vi "TimeTracker_GV.vi"(1 "Action":T1, 2 "Element In":T2) -> (6 "Elements Out":T2[](array[typedef]))   [LabVIEW 2014]
uses:
  Element.ctl
  States.ctl
panel:
  out "Init?":bool
  out "Error Out":errorcluster
  in  "Error In":errorcluster
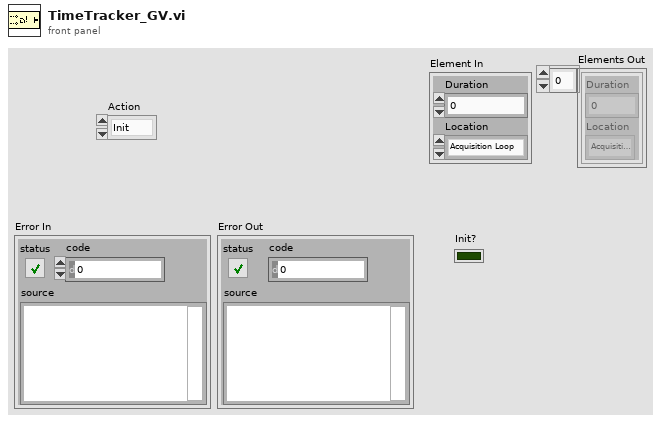
[diagram p1: front panel]
types:
  T1 = typedef "States.ctl" = enum16{"Init", "Flush", "Add"}
  T2 = typedef "Element.ctl" = cluster{"Duration":dbl, "Location":enum16{"Acquisition Loop", "VISA Loop", "FFT Loop", "Spectrogram Loop"}}
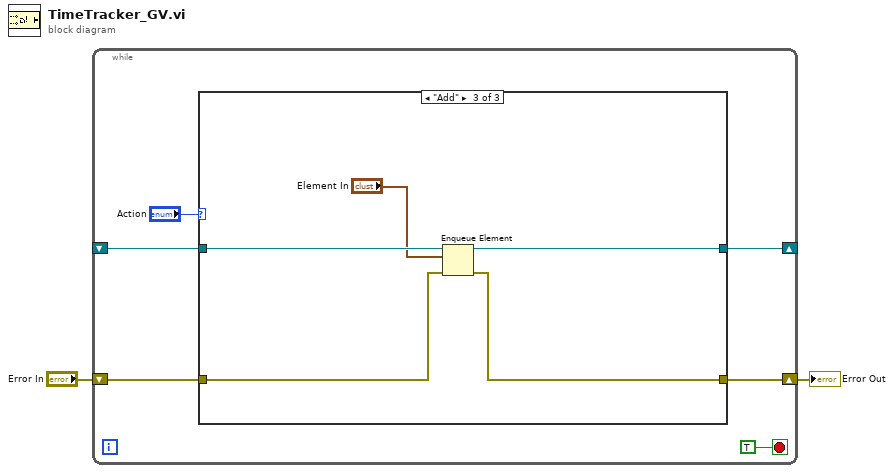
[diagram p0: block diagram]
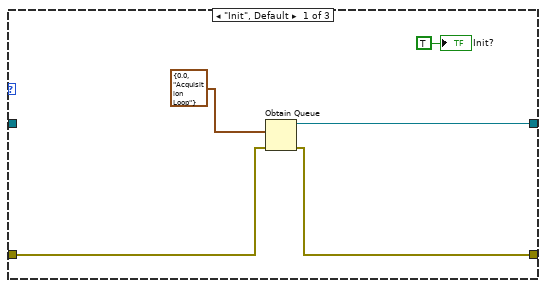
[diagram p2: hidden frame]
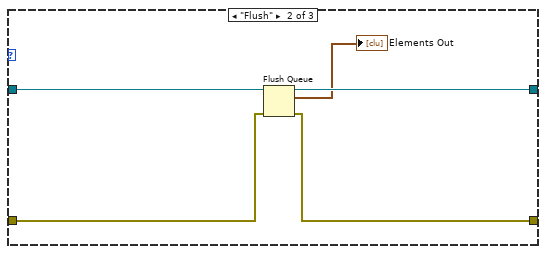
[diagram p3: hidden frame]
diagram:
  n1 = while {
    shift-right: [w7] -> _
    shift-left: _ -> [w6]
    shift-right: [w5] -> w1
    shift-left: "Error In" -> [w4]
    stop <- TRUE stop-if-true
    n2 = case shown="\"Add\"" "Action" {
      tunnel: [w13 w15 w22] -> w7
      tunnel: w6 -> [_ w16 w23]
      tunnel: [w11 w17 w19] -> w5
      tunnel: w4 -> [w10 w18 w20]
      frame "Init", Default {
        n3 = Obtain Queue(element data type=T2 {"Duration"=0.0, "Location"=enum."Acquisition Loop"}, error in (no error)=w10) -> (queue out=w13:refnum<queue>, error out=w11:errorcluster)  [unwired: 3 in, 1 out]
        "Init?" <- TRUE ("Init?")
      }
      frame "Flush" {
        n4 = Flush Queue(queue=w16, error in (no error)=w18) -> (queue out=w15:refnum<queue>, remaining elements=→"Elements Out":T2[], error out=w17:errorcluster)
      }
      frame "Add" {
        n5 = Enqueue Element(queue=w23, element="Element In", error in (no error)=w20) -> (queue out=w22:refnum<queue>, error out=w19:errorcluster)  [unwired: 1 in, 1 out]
      }
    }
  }
  "Error Out" <- w1
